vi "Call The Create Error VI Creator Project.vi"(8 "error in":errorcluster, 11 "Project in":refnum<class "Project.lvclass">) -> (0 "error out":errorcluster)   [LabVIEW 2020, in "Panther Dashboard.lvlib"]
uses:
  Panther Dashboard.lvlib
  Class/Project/Project.lvclass
  <vilib>/PantherLAB/Panther Constants and Errors/Libraries/ConstantErrorsMaker/Selection Info--cluster.ctl
  <vilib>/PantherLAB/Panther Constants and Errors/Libraries/ConstantErrorsMaker/Selection Type--enum.ctl
  Calling mode--enum.ctl
  Class/Library/Library.lvclass/Library.ctl
  Class/LabVIEWItem/LabVIEWItem.lvclass/LabVIEWItem.ctl
  Class/Project/Project.lvclass/Project.ctl
  Class/LabVIEWItem/Read Item Tag.vi
  Class/Library/Read Library Ref.vi
  Class/LabVIEWItem/Read Item Path.vi
  Class/Library/Read Type.vi
  Class/Project/Read Project Ref.vi
  Class/Project/Read Main App Inst Ref.vi
  <vilib>/PantherLAB/Panther Constants and Errors/Libraries/ConstantErrorsMaker/PantherLAB_lib_ConstantErrorsMaker.lvlib
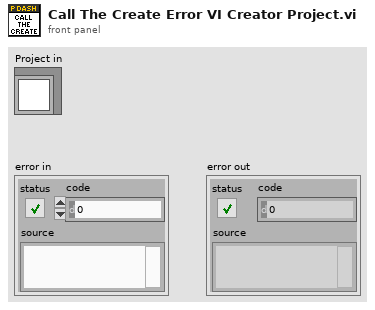
[diagram p1: front panel]
types:
  T1 = typedef "Panther Dashboard.lvlib/Calling mode--enum.ctl" = enum16{"Call and Forguet", "Call and Collect"}
  T2 = typedef "PantherLAB_lib_ConstantErrorsMaker.lvlib/Selection Type--enum.ctl" = enum16{"Project", "Library", "Class", "DQMH Singleton", "DQMH Cloneable"}
  T3 = typedef "PantherLAB_lib_ConstantErrorsMaker.lvlib/Selection Info--cluster.ctl" = cluster{"Name":string, "Library Ref":refnum<vi>, "Application Instance":refnum<vi>, "Selection Owning Folder":path, "Selection Type":T2, "Project Reference":refnum<vi>, "LVClassLibrary Refnum":refnum<vi>}
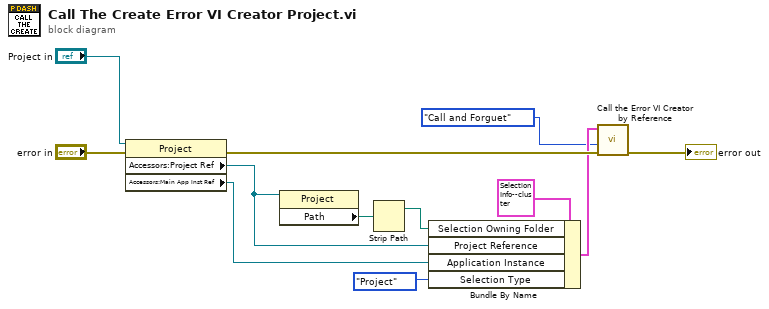
[diagram p0: block diagram]
diagram:
  n1 = property class="Project"(reference="Project in", error in="error in") -> (error out=w11:errorcluster, "Accessors:Project Ref"=w3:refnum<vi>, "Accessors:Main App Inst Ref"=w8:refnum<vi>)  [unwired: 1 out]
  n2 = property class="Project"(reference=w3) -> ("Path"=w2:path)  [unwired: 1 in, 2 out]
  n3 = Strip Path(path=w2) -> (stripped path=w1:path)  [unwired: 1 out]
  n4 = Bundle By Name(cluster=T3 {"Name"="", "Library Ref"=refnum, "Application Instance"=refnum, "Selection Owning Folder"=path "", "Selection Type"=enum."Project", "Project Reference"=refnum, "LVClassLibrary Refnum"=refnum} ("Selection"), "Selection Owning Folder"=w1, "Project Reference"=w3, "Application Instance"=w8, "Selection Type"=Selection_Type--enum."Project") -> (w7:T3)
  n5 = call "Call the Error VI Creator by Reference.vi"("error in"=w11, "Calling mode"=Calling_mode--enum."Call and Forguet", "Selection"=w7) -> ("error out"=→"error out":errorcluster)  [unwired: 6 in, 2 out]
